vi "Stop.vi"() -> ()   [LabVIEW 2010]
panel:
  in  "stop":bool
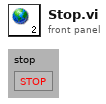
[diagram p1: front panel]
diagram:
